vi "SVFA FFT Spectrum Subset (Real-Im) (N Ch).vi"(0 "scaled signals [EU]":waveform(dbl)[](array[waveform]), 2 "window":T1=1 items=["None"=0, "Hanning"=1, "Hamming"=2, "Blackman-Harris"=3, "Exact Blackman"=4, "Blackman"=5, "Flat Top"=6, "4 Term B-Harris "=7, "7 Term B-Harris"=8, "Low Sidelobe"=9, "Force"=64, "Exponential"=65, "Blackman Nuttall"=11, "Triangle"=30, "Bartlett-Hanning"=31, "Bohman"=32, "Parzen"=33, "Welch"=34, "Kaiser"=60, "Dolph-Chebyshev"=61, "Gaussian"=62], 3 "frequency range":T3={"start frequency"=1000.0, "stop frequency"=5000.0} {"stop frequency" min=0.0 format="%.2f"; "start frequency" min=0.0 format="%.2f"}, 5 "error in (no error)":errorcluster, 7 "averaging parameters":T10={"averaging mode"=enum."No averaging", "weighting mode"=enum."Exponential", "number of averages"=10, "linear mode"=enum."One shot"} {"number of averages" min=1 step=1}, 9 "restart averaging (F)":bool) -> (11 "averaging done":bool, 13 "averages completed":dbl, 14 "real parts [EU rms]":cluster{"f0":dbl, "df":dbl, "real part":dbl[]}[](array[cluster]) {"real part" format="%.2p"; "df" format="%.2p"; "f0" format="%.2p"}, 16 "imaginary parts [EU rms]":T2(array[cluster]) {"imaginary part" format="%.2p"; "df" format="%.2p"; "f0" format="%.2p"}, 17 "unit labels":string[](array[string]), 18 "spectrum info":T4[](array[typedef]) {"x-axis units" items=["Time (s)"=0, "Frequency-CB (Hz)"=1, "Frequency-CPB (Hz)"=1248, "Frequency-Arbitrary (Hz)"=2357, "Quefrency (s)"=2, "Revolutions (rev)"=3, "Order"=4, "Speed (RPM)"=11, "Speed (rad/s)"=21, "Index"=65535]; "weighting filter" items=["Linear", "A-weighting", "B-weighting", "C-weighting", "ITU-R 468-4", "Dolby", "CCITT", "C-message", "Wb", "Wc", "Wd", "We", "Wf", "Wh", "Wj", "Wk", "Wm", "AES17 20 kHz lowpass", "AES17 40 kHz lowpass", "AES17 20 kHz highpass", "AES17 40 kHz highpass"]; "dB reference [EU]" format="%.2f"; "engineering units" items=["custom..."=0, "V"=1, "A"=21, "C"=30, "pC"=31, "s"=32, "-"=29, "Pa"=2, "N"=20, "g"=3, "m/s^2"=4, "m/s"=5, "m"=6, "mm/s"=12, "mm"=13, "micron/s"=14, "micron"=15, "in/s^2"=7, "in/s"=8, "in"=9, "mil/s"=10, "mil"=11, "rad/s^2"=16, "rad/s"=17, "rad"=18, "deg/s^2"=26, "deg/s"=27, "deg"=28, "RPM"=22, "cycle/s^2"=23, "Hz"=24, "cycle"=25, "strain"=19]; "spectral info"."window" items=["None "=0, "Hanning"=1, "Hamming"=2, "Blackman-Harris"=3, "Exact Blackman"=4, "Blackman"=5, "Flat Top"=6, "4 Term B-Harris "=7, "7 Term B-Harris"=8, "Low Sidelobe"=9, "Force - Exponential"=10, "Gaussian"=62]}, 19 "error out":errorcluster)   [LabVIEW 2017]
doc: "Computes a subset of the FFT spectrum of <B>scaled signal [EU]</B>. The subset is defined by <B>frequency range</B>. FFT results are returned as real part and imaginary part. Each block of data corresponds to a single FFT block and has to be passed individually to the this VI. Wire data to the <B>scaled signal [EU]</B> input to determine the polymorphic instance to use or manually select the instance."
uses:
  <vilib>/addons/_NISVFA/_Shared subVIs/Controls/svc_Spectrum Info.ctl
  <vilib>/addons/_NISVFA/_Shared subVIs/Controls/svc_X-Axis Units.ctl
  <vilib>/addons/_NISVFA/_Shared subVIs/Controls/svc_Spectrum Type.ctl
  <vilib>/addons/_NISVFA/_Shared subVIs/Controls/svc_Engineering Units Text Ring.ctl
  <vilib>/addons/_NISVFA/_Shared subVIs/Controls/svc_Weighting Filter Text Ring.ctl
  <vilib>/addons/_NISVFA/_Shared subVIs/Controls/svc_Complimentary Spectrum Units.ctl
  <vilib>/addons/_NISVFA/_Shared subVIs/Controls/svc_Window.ctl
  <vilib>/addons/_NISVFA/_Shared subVIs/Windowing/svfa_Scaled Time Domain Window (1 Ch).vi
  <vilib>/addons/_NISVFA/_Shared subVIs/Spectrum Info/svfa_Build Spectrum Info.vi
  <vilib>/addons/_NISVFA/_Shared subVIs/Spectrum Averaging/svfa_Reset Averaging State Info.vi
  <vilib>/addons/_NISVFA/_Shared subVIs/Spectrum Averaging/svfa_Average Array with Avg Checks (complex) No State.vi
  <vilib>/addons/_NISVFA/_Shared subVIs/Common/svc_Complex to Mag2 Array.vi
  <vilib>/addons/_NISVFA/_Shared subVIs/Spectrum Averaging/svfa_Average Array with Avg Checks (real) No State.vi
  <vilib>/addons/_NISVFA/_Shared subVIs/Windowing/svfa_Scaled Time Domain Window (Array).vi
  <vilib>/addons/_NISVFA/_Shared subVIs/Common/svc_Get SV Channel Info.vi
  <vilib>/addons/_NISVFA/_Shared subVIs/Common/svc_Spectrum Units.vi
  <vilib>/addons/_NISVFA/_Shared subVIs/Spectrum Averaging/svfa_Average Array (complex) No State.vi
  <vilib>/addons/_NISVFA/_Shared subVIs/Spectrum Averaging/svfa_Average Array (real) No State.vi
  <vilib>/Analysis/4window.llb/Force Window.vi
  <vilib>/Analysis/4window.llb/Force Window (DBL).vi
  <vilib>/Analysis/4window.llb/Exponential Window.vi
  <vilib>/Analysis/4window.llb/Exponential Window (DBL).vi
  <vilib>/addons/_NISVFA/_Shared subVIs/Spectrum Averaging/svfa_No Average Array (complex).vi
  <vilib>/addons/_NISVFA/_Shared subVIs/Spectrum Averaging/svfa_Average Array (complex).vi
  <vilib>/addons/_NISVFA/_Shared subVIs/Spectrum Averaging/svfa_No Average Array (real).vi
  <vilib>/addons/_NISVFA/_Shared subVIs/Spectrum Averaging/svfa_Average Array (real).vi
  <vilib>/addons/_NISVFA/_Shared subVIs/Spectrum Averaging/svfa_Peak Hold Array.vi
  <vilib>/addons/_NISVFA/_Shared subVIs/Common/svc_Get Weighting Enum and Labels.vi
  <vilib>/addons/_NISVFA/_Shared subVIs/Common/svc_Unit Label Lexical Class.vi
  <vilib>/addons/_NISVFA/_Shared subVIs/Common/svc_Engineering Units to Unit Label.vi
  <vilib>/addons/_NISVFA/_Shared subVIs/Common/svc_Format Value (DBL).vi
  <vilib>/addons/_NISVFA/_Shared subVIs/Common/svc_Channel Info to Spectrum Info.vi
  <vilib>/addons/_NISVFA/_Shared subVIs/Common/svc_Unit Label to Engineering Units.vi
  <vilib>/Utility/error.llb/Error Cluster From Error Code.vi
  <vilib>/Analysis/0measdsp.llb/Scaled Time Domain Window.vi
  <vilib>/Analysis/0measdsp.llb/Scaled Time Domain Window (DBL).vi
  <vilib>/addons/_NISVFA/_Spectrum Processing/subVIs/svfa_Spectrum Info Window to windowTd Type Def.vi
  <vilib>/addons/_NISVFA/_Shared subVIs/Common/svc_Window Parameters.vi
  <vilib>/addons/_NISVFA/_Shared subVIs/Common/svc_Get Window Info.vi
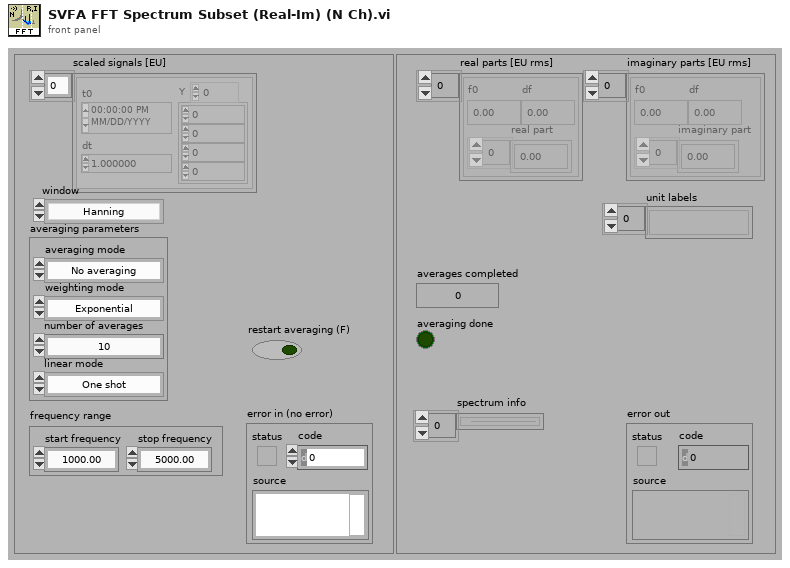
[diagram p1: front panel]
types:
  T1 = typedef "svc_Window.ctl" = u32
  T2 = cluster{"f0":dbl, "df":dbl, "imaginary part":dbl[]}[]
  T3 = cluster{"start frequency":dbl, "stop frequency":dbl}
  T4 = typedef "svc_Spectrum Info.ctl" = cluster{"channel name":string, "description":string, "x-axis units":T5, "spectral info":cluster{"spectrum type":T6, "linear/dB":enum16{"linear", "dB"}, "window":u16, "window size":i32, "FFT size":i32}, "engineering units":T7, "custom label":string, "dB reference [EU]":dbl, "peak units":enum16{"rms", "peak", "peak-peak"}, "weighting filter":T8, "spectral density?":bool, "unit label":string, "spectrum skewed?":bool, "complimentary spectrum units":T9}
  T5 = typedef "svc_X-Axis Units.ctl" = u16
  T6 = typedef "svc_Spectrum Type.ctl" = enum16{"FFT Spectrum [complex]", "Amplitude [Magnitude]", "Power [Magnitude^2]", "Cross Spectrum [complex]", "Frequency Response [Complex]"}
  T7 = typedef "svc_Engineering Units Text Ring.ctl" = u16
  T8 = typedef "svc_Weighting Filter Text Ring.ctl" = u16
  T9 = typedef "svc_Complimentary Spectrum Units.ctl" = enum16{"none", "radians", "degrees", "cycles", "imaginary"}
  T10 = cluster{"averaging mode":enum16{"No averaging", "Vector averaging", "RMS averaging", "Peak hold"}, "weighting mode":enum16{"Linear", "Exponential"}, "number of averages":u32, "linear mode":enum16{"One shot", "Auto restart"}}
  T11 = enum16{"Restart processing", "Continue processing", "Skip processing"}
  T12 = cluster{"complex FFT":cdb[], "real FFT":dbl[], "f0":dbl, "df":dbl, "averages completed":dbl, "averaging parameters":cluster{"averaging mode":enum16{"No averaging", "Vector averaging", "RMS averaging", "Peak hold"}, "weighting mode":enum16{"Linear", "Exponential"}, "number of averages":u32, "linear mode":enum16{"One shot", "Auto restart"}}}
  T13 = cluster{"complex FFT":cdb[], "real FFT":dbl[], "f0":dbl, "df":dbl, "averages completed":dbl, "averaging parameters":cluster{"averaging mode":enum16{"No averaging", "Vector averaging", "RMS averaging", "Peak hold"}, "weighting mode":enum16{"Linear", "Exponential"}, "number of averages":u32, "linear mode":enum16{"One shot", "Auto restart"}}}[]
  T14 = enum16{"No averaging", "Vector averaging", "RMS averaging", "Peak hold"}
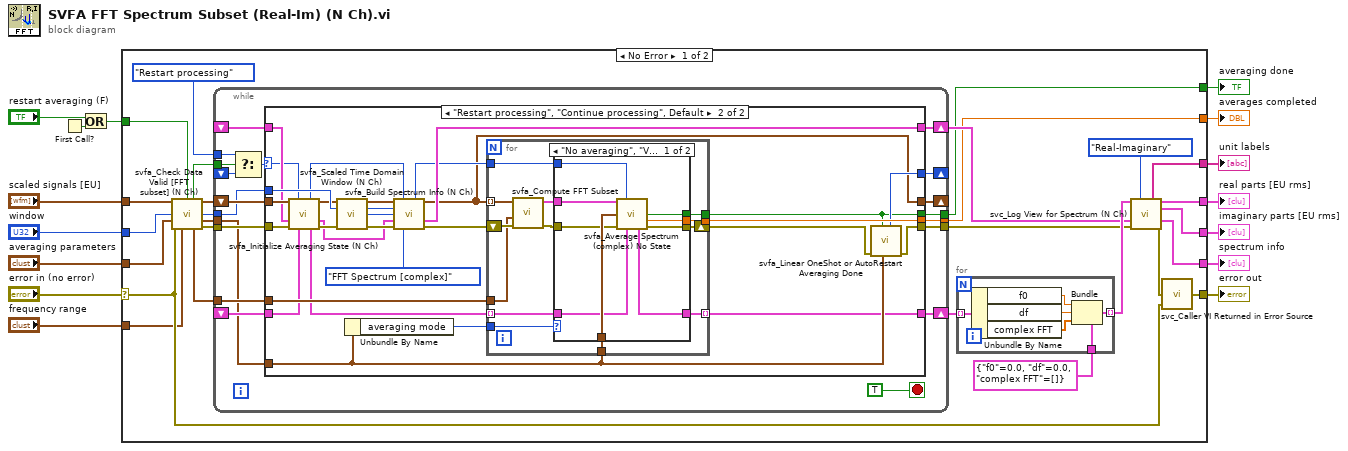
[diagram p0: block diagram]
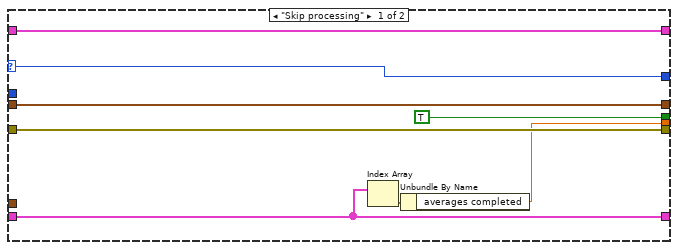
[diagram p2: hidden frame]
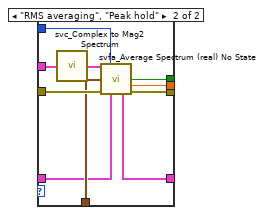
[diagram p3: hidden frame]
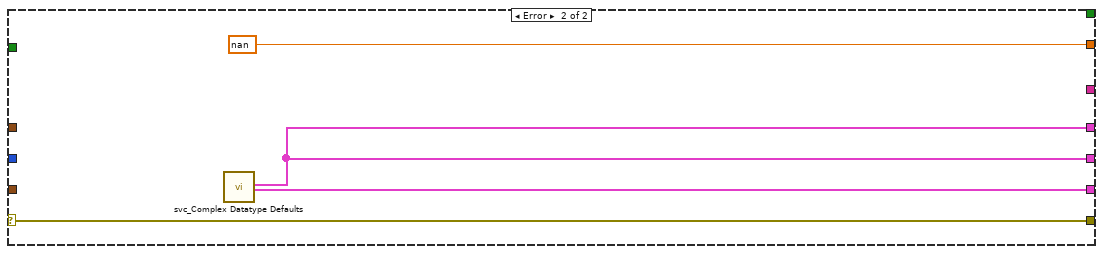
[diagram p4: hidden frame]
diagram:
  n1 = First Call?() -> (First Call?: T/F=w5:bool)
  n2 = Or(x="restart averaging (F)", y=w5) -> (x .or. y?=w3:bool)
  n3 = case shown="No Error" "error in (no error)" {
    selector: "error in (no error)" -> [w33 w140]
    tunnel: w3 -> [w39 _]
    tunnel: [w17 nan ("Averaged So-far")] -> w15
    tunnel: [w34 w140] -> w14
    tunnel: "averaging parameters" -> [w40 _]
    tunnel: "frequency range" -> [w30 _]
    tunnel: "scaled signals [EU]" -> [w42 _]
    tunnel: [w35 w137] -> w6
    tunnel: [w41 _] -> w1
    tunnel: [w37 w138] -> w9
    tunnel: [w38 w138] -> w8
    tunnel: [w16 _] -> w7
    tunnel: "window" -> [w32 _]
    frame No Error {
      n4 = call <vilib>:"svfa_Check Data Valid [FFT subset] (N Ch).vi"("scaled signals"=w42, "restart averaging (F)"=w39, "window"=w32, "averaging parameters"=w40, "error in (no error)"=w33, "frequency range in"=w30) -> ("restart averaging"=w21:bool, "dup scaled signals"=w26:waveform(dbl)[], "window"=w25:u16, "dup averaging parameters"=w24:T10, "frequency range out"=w22:T3, "error out"=w23:errorcluster)  [unwired: 4 in]
      n5 = while {
        shift-left: _ -> [w59]
        shift-right: [w60] -> w29
        tunnel: w22 -> [w62]
        tunnel: [w64] -> w17
        tunnel: [w66] -> w16
        tunnel: w23 -> [w67]
        tunnel: [w65] -> w18
        tunnel: w25 -> [w55]
        tunnel: w24 -> [w54]
        shift-right: [w57] -> w19
        shift-left: _ -> [w56]
        shift-right: [w61] -> _
        shift-left: _ -> [w53]
        tunnel: T11."Restart processing" ("t") -> [w52]
        tunnel: w21 -> [w50]
        shift-right: [w49] -> _
        shift-left: w26 -> [w63]
        stop <- TRUE stop-if-true
        n6 = Select(t=w52, s=w50, f=w53) -> (s? t:f=w51:T11)
        n7 = case shown="\"Restart processing\", \"Continue processing\", Default" w51 {
          selector: w51 -> [w73 w78]
          tunnel: w54 -> [_ w102]
          tunnel: [w72 w96] -> w60
          tunnel: w63 -> [w68 w86]
          tunnel: w62 -> [_ w88]
          tunnel: [w73 w101] -> w61
          tunnel: w59 -> [w72 w83]
          tunnel: w55 -> [_ w103]
          tunnel: [w69 w89] -> w57
          tunnel: w56 -> [w69 w85]
          tunnel: [TRUE ("averaging done?") w98] -> w66
          tunnel: [w70 w104] -> w64
          tunnel: [w74 w100] -> w65
          tunnel: w67 -> [w74 w81]
          tunnel: [w68 w76] -> w49
          frame "Skip processing" {
            n8 = Index Array(array=w72) -> (element=w71:T12)  [unwired: 1 in]
            n9 = Unbundle By Name(w71) -> ("averages completed"=w70:dbl)
          }
          frame "Restart processing", "Continue processing", Default {
            n10 = call <vilib>:"svfa_Initialize Averaging State (N Ch).vi"("Windowed Waveform(s)"=w86, "processing control in"=w78, "spectra info in"=w85, "error in (no error)"=w81, "state info"=w83) -> ("processing control out"=w77:T11, "Windowed Waveform(s)"=w84:waveform(dbl)[], "spectra info out"=w79:T4[], "state info"=w82:T13, "error out"=w80:errorcluster)  [unwired: 6 in]
            n11 = call <vilib>:"svfa_Scaled Time Domain Window (N Ch).vi"("Scaled signal(s)"=w84, "window"=w103, "error in (no error)"=w80) -> ("Windowed Waveform(s)"=w93:waveform(dbl)[], "window"=w91:T1, "window length"=w92:i32, "error out"=w94:errorcluster)  [unwired: 8 in, 1 out]
            n12 = Unbundle By Name(w102) -> ("averaging mode"=w97:T14)
            n13 = call <vilib>:"svfa_Build Spectrum Info (N Ch).vi"("scaled signal(s)"=w93, "processing control in"=w77, "window"=w91, "window size"=w92, "spectra info in"=w79, "error in (no error)"=w94, "spectrum type"=svc_Spectrum_Type."FFT Spectrum [complex]" ("spectrum type 2")) -> ("dup processing control"=w87:T11, "dup scaled signals"=w76:waveform(dbl)[], "spectra info out"=w89:T4[], "error out"=w95:errorcluster)  [unwired: 5 in]
            n14 = for {
              tunnel: [w117] -> w104
              tunnel: w102 -> [w116]
              tunnel: [w114] -> w98
              tunnel: w97 -> [w113]
              tunnel: [w112] -> w96 mode=indexing
              tunnel: w88 -> [w110]
              tunnel: w87 -> [w107]
              tunnel: w76 -> [w106] mode=indexing
              tunnel: w82 -> [w105] mode=indexing
              shift-right: [w115] -> w99
              shift-left: w95 -> [w111]
              n15 = call <vilib>:"svfa_Compute FFT Subset.vi"("error in (no error)"=w111, "frequency range"=w110, "windowed signal"=w106) -> ("error out"=w109:errorcluster, "FFT spectrum [Vrms]"=w108:cluster{"f0":dbl, "df":dbl, "spectrum":cdb[]})  [unwired: 7 in]
              n16 = case shown="\"No averaging\", \"Vector averaging\"" w113 {
                tunnel: w116 -> [w125 w133]
                tunnel: [w123 w129] -> w115
                tunnel: [w122 w135] -> w114
                tunnel: w108 -> [w126 w130]
                tunnel: w109 -> [w124 w136]
                tunnel: [w120 w134] -> w117
                tunnel: w107 -> [w121 w131]
                tunnel: [w119 w127] -> w112
                tunnel: w105 -> [w118 w128]
                frame "No averaging", "Vector averaging" {
                  n17 = call <vilib>:"svfa_Average Spectrum (complex) No State.vi"("spectrum"=w126, "processing control"=w121, "averaging parameters"=w125, "error in (no error)"=w124, "averaging state info in"=w118) -> ("averaging done"=w122:bool, "averages completed"=w120:dbl, "averaging state info out"=w119:T12, "error out"=w123:errorcluster)  [unwired: 5 in, 2 out]
                }
                frame "RMS averaging", "Peak hold" {
                  n18 = call <vilib>:"svc_Complex to Mag2 Spectrum.vi"("complex spectrum"=w130) -> ("power spectrum"=w132:cluster{"f0":dbl, "df":dbl, "spectrum":dbl[]})  [unwired: 4 in]
                  n19 = call <vilib>:"svfa_Average Spectrum (real) No State.vi"("spectrum"=w132, "processing control"=w131, "averaging parameters"=w133, "error in (no error)"=w136, "averaging state info in"=w128) -> ("averaging done"=w135:bool, "averages completed"=w134:dbl, "averaging state info out"=w127:T12, "error out"=w129:errorcluster)  [unwired: 5 in, 2 out]
                }
              }
            }
            n20 = call <vilib>:"svfa_Linear OneShot or AutoRestart Averaging Done.vi"("averaging parameters"=w102, "averaging done"=w98, "error in (no error)"=w99) -> ("error out"=w100:errorcluster, "processing control"=w101:T11)  [unwired: 7 in]
          }
        }
      }
      n21 = for {
        tunnel: w29 -> [w45] mode=indexing
        tunnel: [w44] -> w20 mode=indexing
        tunnel: cluster{"f0":dbl, "df":dbl, "complex FFT":cdb[]} {"f0"=0.0, "df"=0.0, "complex FFT"=[]} ("cluster") -> [w43]
        n22 = Unbundle By Name(w45) -> ("f0"=w48:dbl, "df"=w47:dbl, "complex FFT"=w46:cdb[])
        n23 = Bundle(cluster=w43, "f0"=w48, "df"=w47, "complex FFT"=w46) -> (w44:cluster{"f0":dbl, "df":dbl, "complex FFT":cdb[]})
      }
      n24 = call <vilib>:"svc_Log View for Spectrum (N Ch).vi"("complex spectra"=w20, "View"=enum16{"Mag-Phase", "Real-Imaginary"}."Real-Imaginary", "spectra info in"=w19, "error in (no error)"=w18) -> ("unit label [mag or real]"=w41:string[], "magnitude or real"=w38:cluster{"f0":dbl, "df":dbl, "magnitude":dbl[]}[], "phase or imaginary"=w37:cluster{"f0":dbl, "df":dbl, "magnitude":dbl[]}[], "spectra info out"=w35:T4[], "error out"=w36:errorcluster)  [unwired: 6 in, 1 out]
      n25 = call <vilib>:"svc_Caller VI Returned in Error Source.vi"("warning input to caller"=w33, "error in (no error)"=w36) -> ("error out"=w34:errorcluster)  [unwired: 3 in]
    }
    frame Error {
      n26 = call <vilib>:"svc_Complex Datatype Defaults.vi"() -> ("empty array of spectra"=w138:cluster{"f0":dbl, "df":dbl, "magnitude":dbl[]}[], "empty array of spectrum info"=w137:T4[])  [unwired: 11 in, 7 out]
    }
  }
  "averages completed" <- w15
  "error out" <- w14
  "spectrum info" <- w6
  "unit labels" <- w1
  "real parts [EU rms]" <- w8
  "imaginary parts [EU rms]" <- w9
  "averaging done" <- w7
